vi "test Encode and Decoding Recursively.vi"() -> ()   [LabVIEW 2020, in "AIM ARINC 664 EncodeDecode.lvclass"]
uses:
  AIM ARINC 664 EncodeDecode.lvclass
  <vilib>/NI/NI VeriStand Encoding and Decoding/Encoding.ctl
  <vilib>/addons/_JKI Toolkits/VI Tester/TestCase.llb/TestCase.lvclass
  <vilib>/NI/NI VeriStand Encoding and Decoding/Encoding and Decoding.lvlib
  C:/Program Files/National Instruments/LabVIEW 2024/vi.lib/addons/_JKI Toolkits/VI Tester/TestCase.llb/TestCase.lvclass
panel:
  out "Message Buffer out":u8[](array[numeric])
  out "Data":u8[](array[numeric])
  out "Array":dbl[](array[numeric])
  out "TestCase out":refnum<class "AIM ARINC 664 EncodeDecode.lvclass">
  in  "TestCase in":refnum<class "AIM ARINC 664 EncodeDecode.lvclass">
  out "error out":errorcluster
  in  "error in (no error)":errorcluster
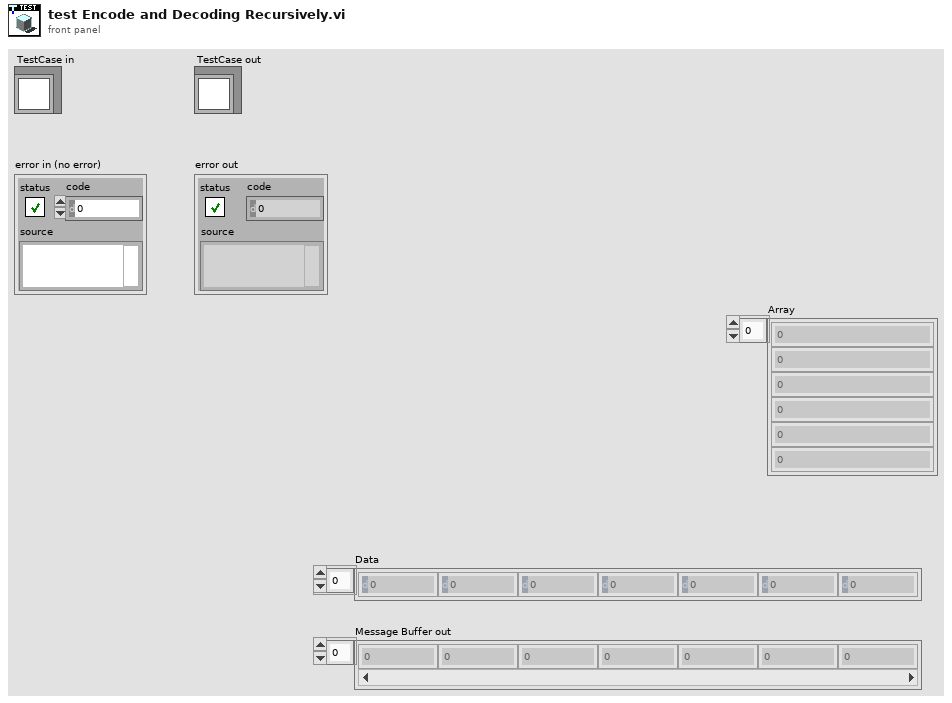
[diagram p1: front panel]
types:
  T1 = typedef "Encoding and Decoding.lvlib/Encoding.ctl" = enum16{"BNR", "BCD", "Discrete"}
  T2 = cluster{"start index":i32, "size":i32, "encoding":T1, "signed":bool, "scale multiplier":dbl, "scale offset":dbl}[]
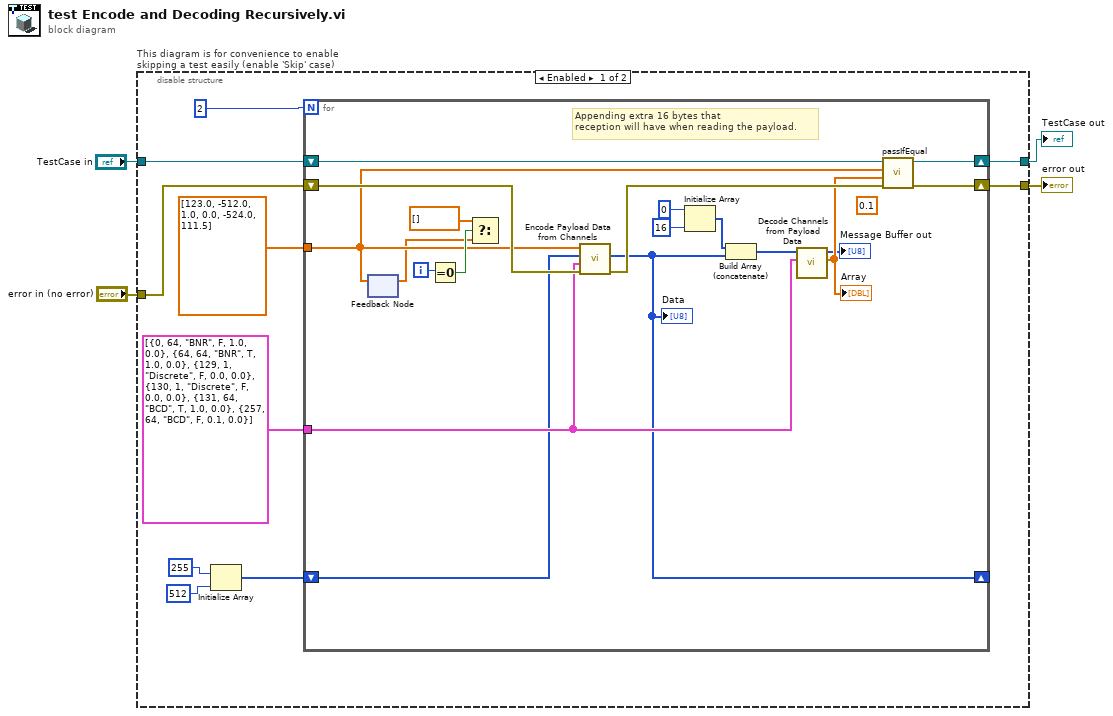
[diagram p0: block diagram]
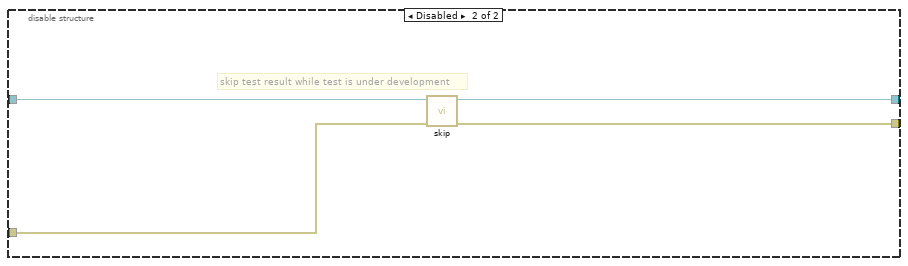
[diagram p2: hidden frame]
diagram:
  n1 = disable-structure "This diagram is for convenience to enable skipping a test easily (enable 'Skip' case)" shown="Enabled" {
    disable-tunnel: "TestCase in" -> [w11 w37]
    disable-tunnel: [w13 w35] -> w2
    disable-tunnel: [w14 w36] -> w3
    disable-tunnel: "error in (no error)" -> [w12 w34]
    frame Enabled {
      n2 = Initialize Array(255 ("dimension size"), 512 ("dimension size")) -> (w5:i32[])
      n3 = for {
        N: 2 ("Numeric") -> [_]
        shift-right: [w33] -> w14
        shift-left: w12 -> [w31]
        shift-right: [w32] -> w13
        shift-left: w11 -> [w30]
        tunnel: dbl[] [123.0, -512.0, 1.0, 0.0, -524.0, 111.5] ("Values in") -> [w18]
        tunnel: T2 [{"start index"=0, "size"=64, "encoding"=enum."BNR", "signed"=FALSE, "scale multiplier"=1.0, "scale offset"=0.0}, {"start index"=64, "size"=64, "encoding"=enum."BNR", "signed"=TRUE, "scale multiplier"=1.0, "scale offset"=0.0}, {"start index"=129, "size"=1, "encoding"=enum."Discrete", "signed"=FALSE, "scale multiplier"=0.0, "scale offset"=0.0}, {"start index"=130, "size"=1, "encoding"=enum."Discrete", "signed"=FALSE, "scale multiplier"=0.0, "scale offset"=0.0}, {"start index"=131, "size"=64, "encoding"=enum."BCD", "signed"=TRUE, "scale multiplier"=1.0, "scale offset"=0.0}, {"start index"=257, "size"=64, "encoding"=enum."BCD", "signed"=FALSE, "scale multiplier"=0.1, "scale offset"=0.0}] ("Parameters") -> [w22]
        shift-right: [w15] -> _
        shift-left: w5 -> [w16]
        i -> [w21]
        (unwired) 0.1 ("Value")
        # "Appending extra 16 bytes that \nreception will have when reading the payload."
        n4 = feedback-in #1(w18) -> ()
        n5 = feedback #1() -> (w17:dbl[])  [unwired: 1 in]
        n6 = Equal To 0?(x=w21) -> (x = 0?=w20:bool)
        n7 = Select(t=dbl[] [], s=w20, f=w17) -> ()  [unwired: 1 out]
        n8 = call "Encode Payload Data from Channels.vi"("error in"=w31, "Parameters"=w22, "Data in"=w16, "Values in"=w18) -> ("error out"=w29:errorcluster, "Data out"=w15:u8[])  [unwired: 5 in, 1 out]
        "Data" <- w15
        n9 = Initialize Array(0 ("element"), 16 ("dimension size")) -> (w24:i32[])
        n10 = Build Array (concatenate)(w24, w15) -> (w23:i32[])
        n11 = call "Decode Channels from Payload Data.vi"("Parameters"=w22, "Message Buffer in"=w23) -> ("Channels"=w28:dbl[], "Message Buffer out"=→"Message Buffer out":u8[])  [unwired: 8 in]
        "Array" <- w28
        n12 = call-dynamic "passIfEqual.vi"("error in (no error)"=w29, "y"=w28, "x"=w18, "TestCase in"=w30) -> ("error out"=w33:errorcluster, "TestCase out"=w32:refnum<class "AIM ARINC 664 EncodeDecode.lvclass">)  [unwired: 6 in]
      }
    }
    frame Disabled {
      # "skip test result while test is under development"
      n13 = call <vilib>:"skip.vi"("error in (no error)"=w34, "TestCase in"=w37) -> ("error out"=w36:errorcluster, "TestCase out"=w35:refnum<class "AIM ARINC 664 EncodeDecode.lvclass">)  [unwired: 8 in]
    }
  }
  "error out" <- w3
  "TestCase out" <- w2
